vi "exmpl_Create_Simulated_Value.vi"(10 "offset":dbl=15.0 format="%#_13g", 11 "seconds since 1Jan1904":timestamp) -> (2 "Numeric":dbl, 3 "Waveform":waveform(dbl))   [LabVIEW 2013, in "daqio minimal.lvlib"]
doc: "This VI creates a simulated value for a temperature or CPU load."
uses:
  daqio minimal.lvlib
  <vilib>/ptbypt/NI_PtbyPt.lvlib
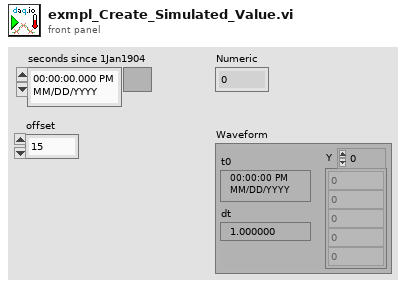
[diagram p1: front panel]
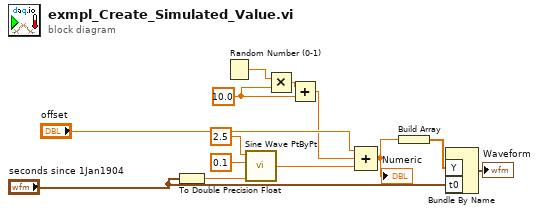
[diagram p0: block diagram]
diagram:
  w3 = 10.0 ("y")
  n1 = To Double Precision Float(number="seconds since 1Jan1904") -> (double precision float=w8:dbl)
  n2 = Random Number (0-1)() -> (number: 0 to 1=w1:dbl)
  n3 = call <vilib>:"Sine Wave PtByPt.vi"("time"=w8, "frequency"=0.1, "amplitude"=2.5) -> ("sine wave"=w9:dbl)  [unwired: 1 in]
  n4 = Multiply(x=w1, y=w3) -> (x*y=w2:dbl)
  n5 = Add(x=w2, y=w3) -> (x+y=w10:dbl)
  n6 = Compound Arithmetic op=ADD("offset", w10, w9) -> (w11:dbl)
  "Numeric" <- w11
  n7 = Build Array(w11) -> (w4:dbl[])
  n8 = Bundle By Name("Y"=w4, "t0"="seconds since 1Jan1904") -> (→"Waveform":waveform(dbl))  [unwired: 1 in]
